vi "create_timetrace_diag.vi"(9 "Boolean":bool, 10 "string":string, 11 "String":string) -> (2 "path":path, 3 "Byte Stream File out":refnum<file>)   [LabVIEW 2013]
uses:
  <vilib>/Utility/file.llb/Write To Spreadsheet File (string).vi
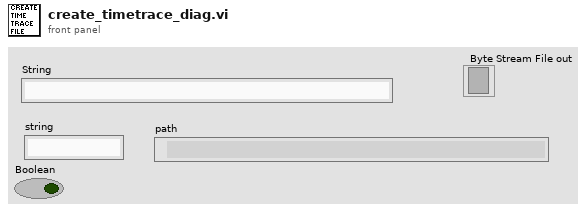
[diagram p1: front panel]
types:
  T1 = enum16{"open", "replace", "create", "open or create", "replace or create", "replace or create with confirmation"}
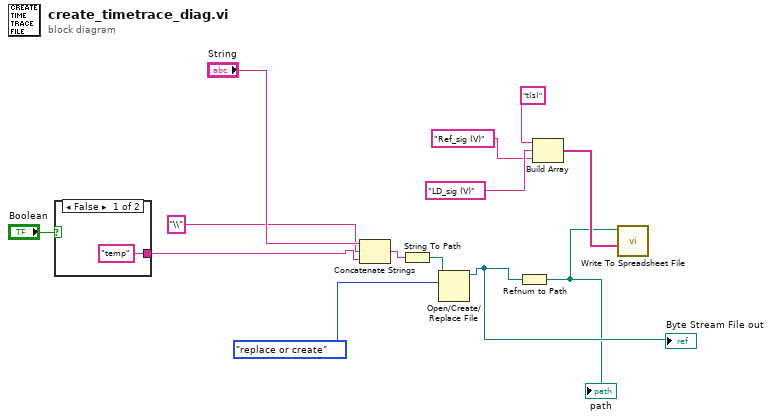
[diagram p0: block diagram]
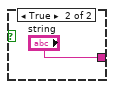
[diagram p2: hidden frame]
diagram:
  n1 = case shown="False" "Boolean" {
    tunnel: ["temp" ("string") "string"] -> w5
    frame False {
    }
    frame True {
    }
  }
  n2 = Concatenate Strings("String", "\\" ("string"), w5) -> (w6:string)
  n3 = String To Path(string=w6) -> (path=w9:path)
  n4 = Open/Create/Replace File(file path (use dialog)=w9, operation (0:open)=T1."replace or create") -> (refnum out=w10:refnum<file>)  [unwired: 4 in, 2 out]
  "Byte Stream File out" <- w10
  n5 = Refnum to Path(1:w10) -> (0:w8:path)
  "path" <- w8
  n6 = Build Array("t(s)" ("element"), "LD_sig (V)" ("element"), "Ref_sig (V)") -> (w13:string[])
  n7 = call-poly <vilib>:"Write To Spreadsheet File.vi"("1D data"=w13, "file path (dialog if empty)"=w8) -> ()  [unwired: 6 in, 1 out]
